vi "Error Code.vi"(6 "Error Code":i32(ring) items=["No error", "Argument error", "Memory is full", "Out of zone", "End of file", "File already open", "Generic file I/O error", "File not found", "File permission error", "Disk is full", "Duplicate path", "Too many files open", "System feature not enabled", "Resource file not found", "Cannot add resource", "Resource not found", "Image not found", "Image memory error", "Pen does not exist", "Config type invalid", "Config token not found", "Config parse error", "Config memory error", "Bad external code format", "Bad external code offset", "External code not present", "Null window", "Destroy window error", "Null menu", "Print aborted", "Bad print record", "Print driver error", "Windows error during printing", "Memory error during printing", "Print dialog error", "Generic print error", "Invalid device refnum", "Device not found", "Device parameter error", "Device unit error", "Cannot open device", "Device call aborted", "Generic error", "Cancelled by user", "Object ID too low", "Object ID too high", "Object not in heap", "Unknown heap", "Unknown object (invalid DefProc)", "Unknown object (DefProc not in table)", "Message out of range", "Invalid (null) method", "Unknown message", "Manager call not supported", "Bad address", "Network operation in progress", "Network operation timed out", "Connection is busy", "Network attribute not supported", "Network error", "Address in use", "System out of memory", "Connection aborted", "Connection refused", "Not connected", "Already connected", "Connection closed", "Initialization error (interapplication manager)", "Bad occurrence", "Wait on unbound occurrence handler", "Occurrence queue overflow", "Datalog type conflict", "Unused", "Unrecognized type (interapplication manager)", "Memory corrupt", "Failed to make temporary DLL", "Old CIN version", "Drag socket not found", "Failed to load drop-object", "Failed to register OLE object", "Failed to release OLE object", "Format specifier type mismatch", "Unknown format specifier", "Too few format specifiers", "Too many format specifiers", "Scan failed", "Newer CIN version", "OLE Convert", "Runtime menu error", "Password tampered", "Unknown error code"], 9 "error in (no error)":errorcluster, 10 "Suppress? (T)":bool=TRUE) -> (1 "error out":errorcluster, 2 "Detected?":bool)   [LabVIEW 2011]
doc: "Checks for error code; optionally clears it.\n\n\nVersion 1.0 - 02/13/2013\n\nPhaeron, Inc.\nwww.phaeron.com\ninfo@phaeron.com"
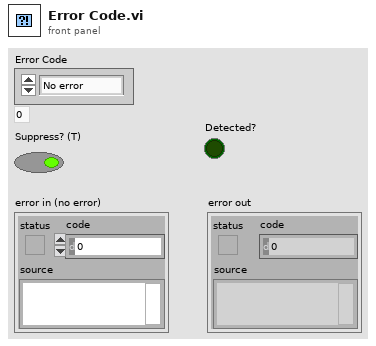
[diagram p1: front panel]
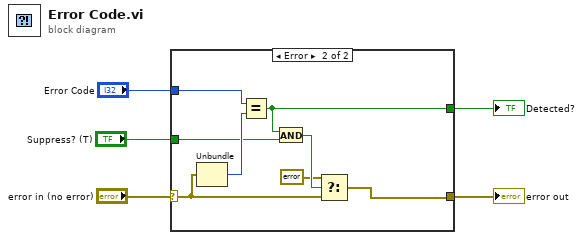
[diagram p0: block diagram]
diagram:
  n1 = case shown="Error" "error in (no error)" {
    selector: "error in (no error)" -> [w6 w7]
    tunnel: [w6 w9] -> w4
    tunnel: "Suppress? (T)" -> [_ w12]
    tunnel: "Error Code" -> [_ w13]
    tunnel: [_ w11] -> w1
    frame No Error {
    }
    frame Error {
      n2 = Unbundle(w7) -> ("code"=w14:i32)  [unwired: 2 out]
      n3 = Equal?(x=w13, y=w14) -> (x = y?=w11:bool)
      n4 = And(x=w11, y=w12) -> (x .and. y?=w10:bool)
      n5 = Select(t=errorcluster {"status"=FALSE, "code"=0, "source"=""}, s=w10, f=w7) -> (s? t:f=w9:errorcluster)
    }
  }
  "error out" <- w4
  "Detected?" <- w1
